vi "Smart Open.vi"(7 "Allow multiple opens?":bool=TRUE, 8 "error in (no error)":errorcluster, 10 "Channel Name":tag) -> (0 "error out":errorcluster, 3 "PWM Ref Out":T1)   [LabVIEW 2021, in "PWM.lvlib"]
uses:
  <vilib>/myRIO/Common/Instrument Driver Framework/Utilities/typedefs/Hardware Version Enum.ctl
  <vilib>/myRIO/Common/Instrument Driver Framework/Utilities/typedefs/Generic FPGA Reference.ctl
  <vilib>/myRIO/Common/Instrument Driver Framework/myRIO v1.0/PWM/typedefs/PWM Channels Enum.ctl
  <vilib>/myRIO/Instrument Drivers/Onboard IO/PWM/typedefs/PWM Configuration.ctl
  <vilib>/myRIO/Instrument Drivers/Onboard IO/PWM/PWM.lvlib
  <vilib>/myRIO/Instrument Drivers/Onboard IO/PWM/typedefs/PWM Reference.ctl
  <vilib>/myRIO/Common/Instrument Driver Framework/Utilities/typedefs/myRIO v1.0 Reference.ctl
  <vilib>/myRIO/Common/Instrument Driver Framework/Utilities/typedefs/myRIO Generic Hardware Reference.ctl
  <vilib>/myRIO/Instrument Drivers/Onboard IO/PWM/vis/myRIO PWM Open.xnode
  <vilib>/myRIO/Common/Instrument Driver Framework/myRIO v1.0/PWM/vis/myRIO v1.1 Open PWM.vi
  <vilib>/userdefined/High Color/nirio_resource_hc.ctl
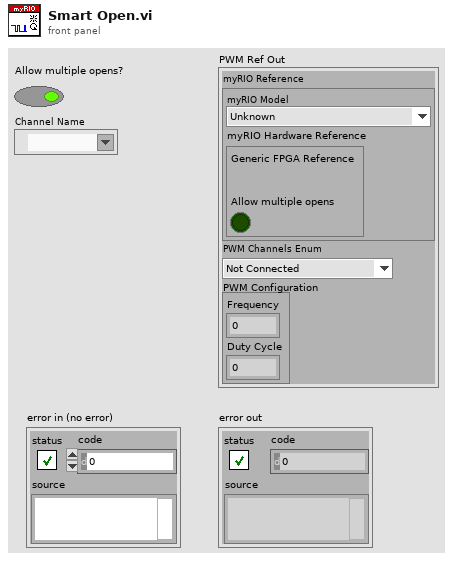
[diagram p1: front panel]
types:
  T1 = typedef "PWM.lvlib/PWM Reference.ctl" = cluster{"myRIO Reference":T2, "PWM Channels Enum":T6, "PWM Configuration":T7}
  T2 = typedef "myRIO Generic Hardware Reference.ctl" = cluster{"myRIO Model":T3, "myRIO Hardware Reference":T4}
  T3 = typedef "Hardware Version Enum.ctl" = enum16{"Unknown", "myRIO-1900", "myRIO-1950", "roboRIO", "NI ELVIS RIO CM", "ELVIS III"}
  T4 = typedef "myRIO v1.0 Reference.ctl" = cluster{"Generic FPGA Reference":T5, "Allow multiple opens":bool}
  T5 = typedef "Generic FPGA Reference.ctl" = refnum<k20>
  T6 = typedef "PWM Channels Enum.ctl" = enum16{"Not Connected", "C/PWM0", "C/PWM1", "A/PWM0", "A/PWM1", "A/PWM2", "A/PWM3", "A/PWM4", "A/PWM5", "A/PWM6", "A/PWM7", "A/PWM8", "A/PWM9", "A/PWM10", "A/PWM11", "A/PWM12", "A/PWM13", "A/PWM14", "A/PWM15", "A/PWM16", "A/PWM17", "A/PWM18", "A/PWM19", "B/PWM0", "B/PWM1", "B/PWM2", "B/PWM3", "B/PWM4", "B/PWM5", "B/PWM6", "B/PWM7", "B/PWM8", "B/PWM9", "B/PWM10", "B/PWM11", "B/PWM12", "B/PWM13", "B/PWM14", "B/PWM15", "B/PWM16", "B/PWM17", "B/PWM18", "B/PWM19", "PWM/PWM0", "PWM/PWM1", "PWM/PWM2", "PWM/PWM3", "PWM/PWM4", "PWM/PWM5", "PWM/PWM6", "PWM/PWM7", "PWM/PWM8", "PWM/PWM9"}
  T7 = typedef "PWM.lvlib/PWM Configuration.ctl" = cluster{"Frequency":dbl, "Duty Cycle":dbl}
  T8 = typedef "nirio_resource_hc.ctl" = tag
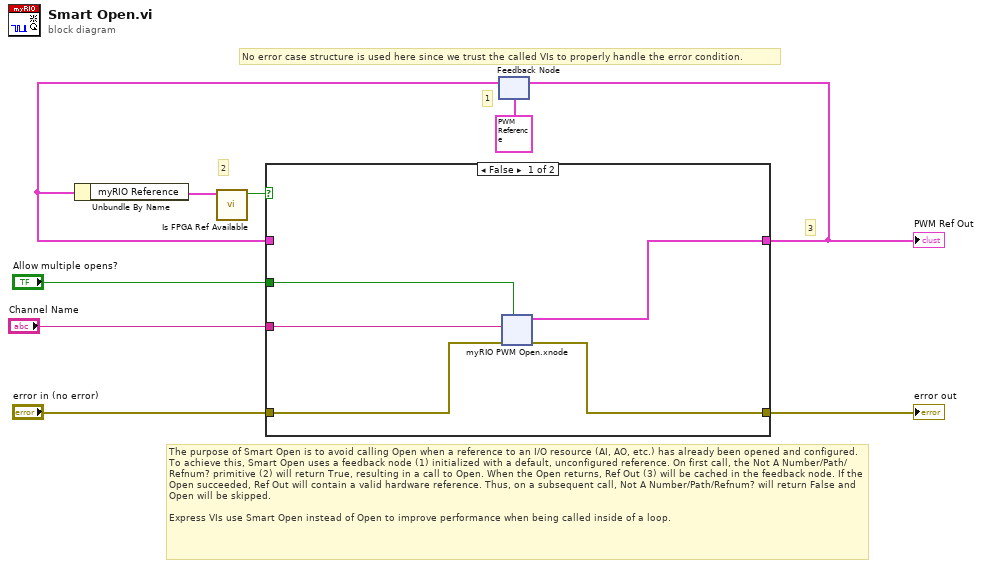
[diagram p0: block diagram]
diagram:
  # "No error case structure is used here since we trust the called VIs to properly handle the error condition."
  # "2"
  # "1"
  # "3"
  # "The purpose of Smart Open is to avoid calling Open when a reference to an I/O resource (AI, AO, etc.) has already been opened and configured. To achieve this, Smart Open uses a feedback node (1) initialized with a default, unconfigured reference. On first call, the Not A Number/Path/Refnum? primitive (2) will return True, resulting in a call to Open. When the Open returns, Ref Out (3) will be cached in the feedback node. If the Open succeeded, Ref Out will contain a valid hardware reference. Thus, on a subsequent call, Not A Number/Path/Refnum? will return False and Open will be skipped.\n\t\nExpress VIs use Smart Open instead of Open to improve performance when being called inside of a loop."
  n1 = feedback #1(T1 {"myRIO Reference"={"myRIO Model"=enum."Unknown", "myRIO Hardware Reference"={"Generic FPGA Reference"=refnum, "Allow multiple opens"=FALSE}}, "PWM Channels Enum"=enum."Not Connected", "PWM Configuration"={"Frequency"=0.0, "Duty Cycle"=0.0}} ("AI Ref Out")) -> (w4:T1)
  n2 = Unbundle By Name(w4) -> ("myRIO Reference"=w1:T2)
  n3 = call <vilib>:"Is FPGA Ref Available.vi"("myRIO Reference"=w1) -> ("Is Available?"=w5:bool)  [unwired: 10 in]
  n4 = case shown="False" w5 {
    tunnel: "error in (no error)" -> [w14 w31]
    tunnel: [w13 w32] -> w7
    tunnel: [w12 w31] -> w8
    tunnel: w4 -> [_ w32]
    tunnel: "Allow multiple opens?" -> [w11 _]
    tunnel: "Channel Name" -> [w10 _]
    frame False {
      n5 = xnode "myRIO PWM Open.xnode"("error in (no error)"=w14, "Allow multiple opens?"=w11, "Channel Name"=w10) -> ("error out"=w12:errorcluster, "PWM Ref Out"=w13:T1)
    }
    frame True {
    }
  }
  "PWM Ref Out" <- w7
  "error out" <- w8
  n6 = feedback-in #1(w7) -> ()
